vi "Set Pane ScrollBars.vi"(7 "Pane Ref":refnum<vi>, 8 "Error":errorcluster, 11 "(FPEN)":refnum<class "(FPEN).lvclass">) -> (0 "Error Out":errorcluster, 3 "(FPEN) Out":refnum<class "(FPEN).lvclass">, 5 "Pane Ref Out":refnum<vi>)   [LabVIEW 2016, in "(FPEN).lvclass"]
uses:
  (FPEN).lvclass
  (FPEN).lvclass/(FPEN).ctl
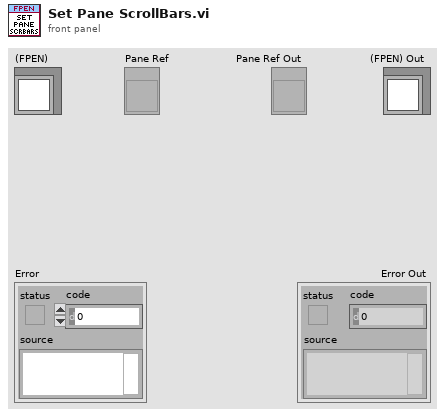
[diagram p1: front panel]
types:
  T1 = typedef "Cluster_FP_Scroll Bars Hide Show.ctl" = cluster{"Horiz SBar":T2, "Vert SBar":T2}
  T2 = typedef "ENUM_FP_Show-Hide Select.ctl" = enum16{"No Change", "Hide", "Show"}
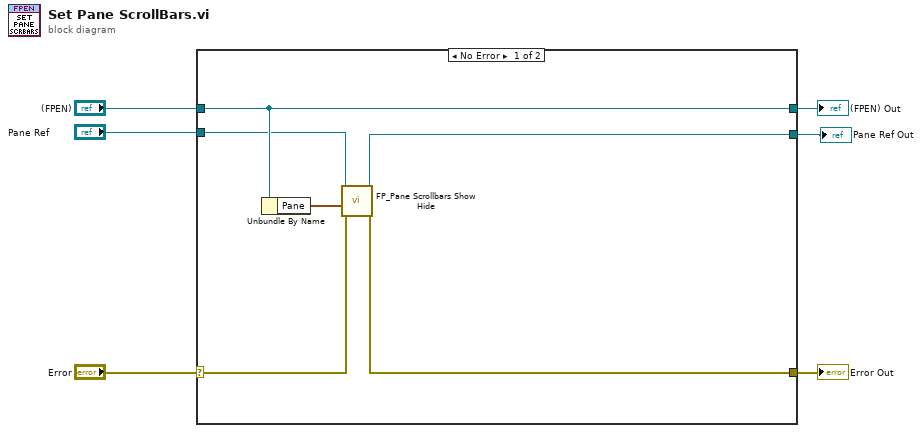
[diagram p0: block diagram]
diagram:
  n1 = case shown="No Error" "Error" {
    selector: "Error" -> [w9 w15]
    tunnel: [w8 w15] -> w5
    tunnel: [w12 w14] -> w3
    tunnel: "(FPEN)" -> [w12 w14]
    tunnel: [w7 w13] -> w2
    tunnel: "Pane Ref" -> [w10 w13]
    frame No Error {
      n2 = Unbundle By Name(w12) -> ("Pane"=w11:T1)
      n3 = call "FP_Pane Scrollbars Show Hide.vi"("Error"=w9, "Scrollbar Settings"=w11, "Pane"=w10) -> ("Error Out"=w8:errorcluster, "Pane Out"=w7:refnum<vi>)  [unwired: 7 in]
    }
    frame Error {
    }
  }
  "Error Out" <- w5
  "(FPEN) Out" <- w3
  "Pane Ref Out" <- w2
